vi "Data Output Format.vi"(6 "Byte Order (Normal)":T1(ring), 8 "error in (no error)":errorcluster, 9 "ASCII Precision (6)":i32=6 min=1 max=16, 10 "Data Format (ASCII)":T2(ring), 11 "VISA resource name":refnum<visa-resource-name>) -> (0 "error out":errorcluster, 3 "VISA resource name out":refnum<visa-resource-name>)   [LabVIEW 2018, in "Keithley 3706.lvlib"]
uses:
  <instrlib>/Keithley 3706/Keithley 3706.lvlib
panel:
  out "Command String":string
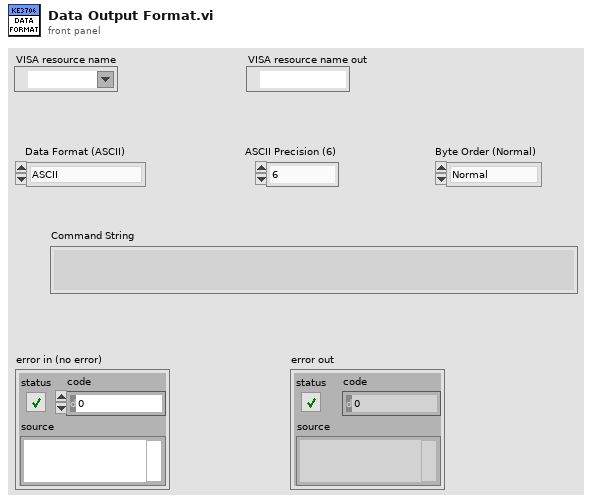
[diagram p1: front panel]
types:
  T1 = enum32{"Normal", "Big Endian", "Little Endian", "Network", "Swapped"}
  T2 = enum32{"ASCII", "Real 32", "Real 64", "Single Precision Real", "Double Precision Real"}
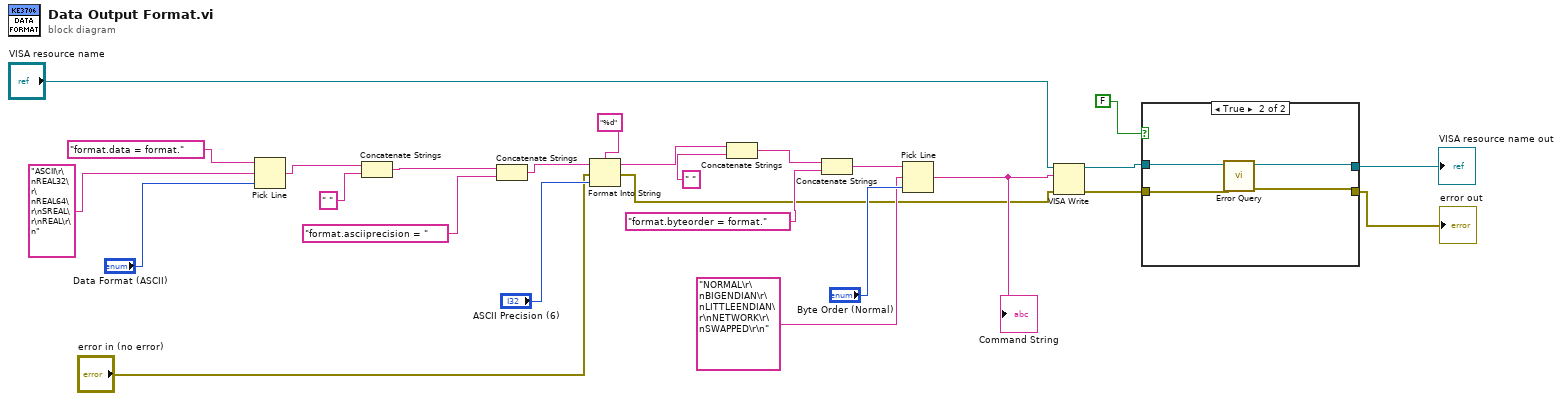
[diagram p0: block diagram]
diagram:
  n1 = Pick Line(string ("")="format.data = format." ("command"), multi-line string="ASCII\r\nREAL32\r\nREAL64\r\nSREAL\r\nREAL\r\n" ("options"), line index="Data Format (ASCII)") -> (output string=w23:string)
  n2 = Concatenate Strings(w23, " " ("command")) -> (w21:string)
  n3 = Concatenate Strings(w21, "format.asciiprecision = " ("command")) -> (w19:string)
  n4 = Format Into String(format string="%d", initial string=w19, error in="error in (no error)", "ASCII Precision (6)") -> (resulting string=w15:string, error out=w7:errorcluster)
  n5 = Concatenate Strings(w15, " " ("command")) -> (w13:string)
  n6 = Concatenate Strings(w13, "format.byteorder = format." ("command")) -> (w11:string)
  n7 = Pick Line(string ("")=w11, multi-line string="NORMAL\r\nBIGENDIAN\r\nLITTLEENDIAN\r\nNETWORK\r\nSWAPPED\r\n" ("options"), line index="Byte Order (Normal)") -> (output string=w8:string)
  "Command String" <- w8
  n8 = VISA Write(VISA resource name="VISA resource name", write buffer=w8, error in (no error)=w7) -> (VISA resource name out=w2:refnum<visa-resource-name>, error out=w5:errorcluster)  [unwired: 1 out]
  n9 = case shown="True" FALSE {
    tunnel: w5 -> [w28 w32]
    tunnel: [w28 w30] -> w3
    tunnel: [w27 w31] -> w1
    tunnel: w2 -> [w27 w29]
    frame False {
    }
    frame True {
      n10 = call <instrlib>:"Error Query.vi"("error in (no error)"=w32, "VISA resource name"=w29) -> ("error out"=w30:errorcluster, "VISA resource name output"=w31:refnum<visa-resource-name>)  [unwired: 6 in, 2 out]
    }
  }
  "VISA resource name out" <- w1
  "error out" <- w3
